vi "Format DateTime Data.vi"(9 "DB String in":string, 10 "Timestamp in":timestamp) -> (1 "Timestamp out":timestamp, 2 "UTC DB String out":string, 5 "NON_UTC String out":string)   [LabVIEW 2011]
uses:
  <vilib>/Utility/miscctls.llb/LVDateTimeRec.ctl
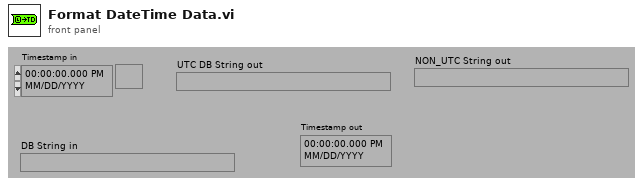
[diagram p1: front panel]
types:
  T1 = typedef "LVDateTimeRec.ctl" = cluster{"fractional second":dbl, "second":i32, "minute":i32, "hour":i32, "day of month":i32, "month":i32, "year":i32, "day of week":i32, "day of year":i32, "DST":i32}
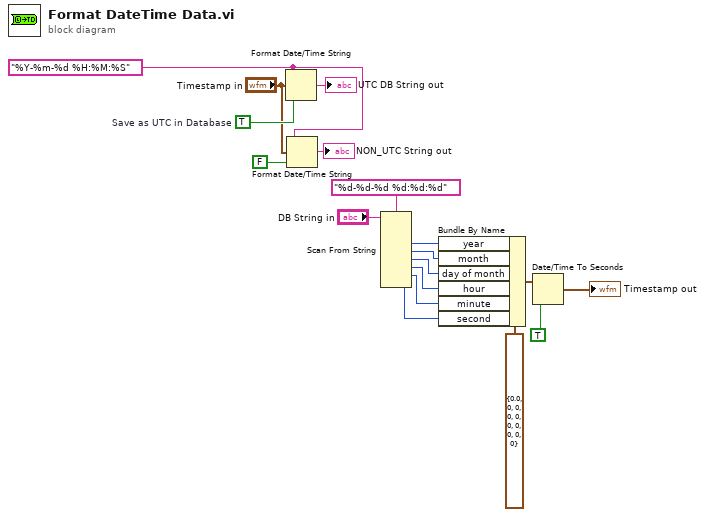
[diagram p0: block diagram]
diagram:
  w18 = TRUE  # Save as UTC in Database
  w1 = "%Y-%m-%d %H:%M:%S" ("time format string (%c)")
  n1 = Format Date/Time String(time format string (%c)=w1, seconds (now)="Timestamp in", UTC format=w18) -> (date/time string=→"UTC DB String out":string)
  n2 = Format Date/Time String(time format string (%c)=w1, seconds (now)="Timestamp in", UTC format=FALSE) -> (date/time string=→"NON_UTC String out":string)
  n3 = Scan From String(format string="%d-%d-%d %d:%d:%d", input string="DB String in") -> (output 1=w11:i32, output 2=w12:i32, output 3=w13:i32, output 4=w14:i32, output 5=w15:i32, output 6=w16:i32)  [unwired: 2 in, 9 out]
  n4 = Bundle By Name(cluster=T1 {"fractional second"=0.0, "second"=0, "minute"=0, "hour"=0, "day of month"=0, "month"=0, "year"=0, "day of week"=0, "day of year"=0, "DST"=0} ("date time rec"), "year"=w11, "month"=w12, "day of month"=w13, "hour"=w14, "minute"=w15, "second"=w16) -> (w17:T1)
  n5 = Date/Time To Seconds(1:TRUE, 2:w17) -> (0:→"Timestamp out":timestamp)
